vi "Periodic Tasks.vi"(8 "error in":errorcluster) -> ()   [LabVIEW 2015]
doc: "This VI runs in parallel to other tasks. It can contain as many user-defined periodic loops as you need. These can carry out PID or other sorts of timed response."
uses:
  <vilib>/Rock Robotics/WPI/Utilities/WPI_GetSetVariantRefNum.vi
  Robot Global Data.vi
  <vilib>/Rock Robotics/Network Tables/SD Write Boolean.vi
  <vilib>/Rock Robotics/Network Tables/SD Write Number.vi
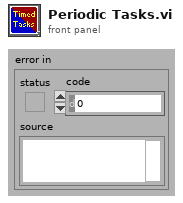
[diagram p1: front panel]
types:
  T1 = typedef "WPI_JoystickDevRef.ctl" = cluster{"Device":T2}
  T2 = typedef "WPI_JoystickDeviceEnum.ctl" = enum16{"USB 0", "USB 1", "USB 2", "USB 3", "USB 4", "USB 5"}
  T3 = cluster{"Axes[0]":dbl, "Axes[1]":dbl, "Axes[2]":dbl, "Axes[3]":dbl, "Axes[4]":dbl, "Axes[5]":dbl, "Axes[6]":dbl, "Axes[7]":dbl, "Axes[8]":dbl}
  T4 = cluster{"Buttons[0]":bool, "Buttons[1]":bool, "Buttons[2]":bool, "Buttons[3]":bool, "Buttons[4]":bool, "Buttons[5]":bool, "Buttons[6]":bool, "Buttons[7]":bool, "Buttons[8]":bool}
  T5 = typedef "WPI_EncoderDevRef.ctl" = cluster{"DevStatus":errorcluster, "EncoderIndex":T6, "CounterIndex":T7, "DistancePerCount":dbl, "Decoding Type":T8}
  T6 = typedef "FPGA_EncoderIdx.ctl" = enum8{"Enc 0", "Enc 1", "Enc 2", "Enc 3", "Enc 4", "Enc 5", "Enc 6", "Enc 7", "Invalid"}
  T7 = typedef "FPGA_CounterCtrSystemIndex.ctl" = enum8{"Ctr 0", "Ctr 1", "Ctr 2", "Ctr 3", "Ctr 4", "Ctr 5", "Ctr 6", "Ctr 7", "Invalid"}
  T8 = typedef "WPI_EncoderType.ctl" = enum16{"1x", "2x", "4x"}
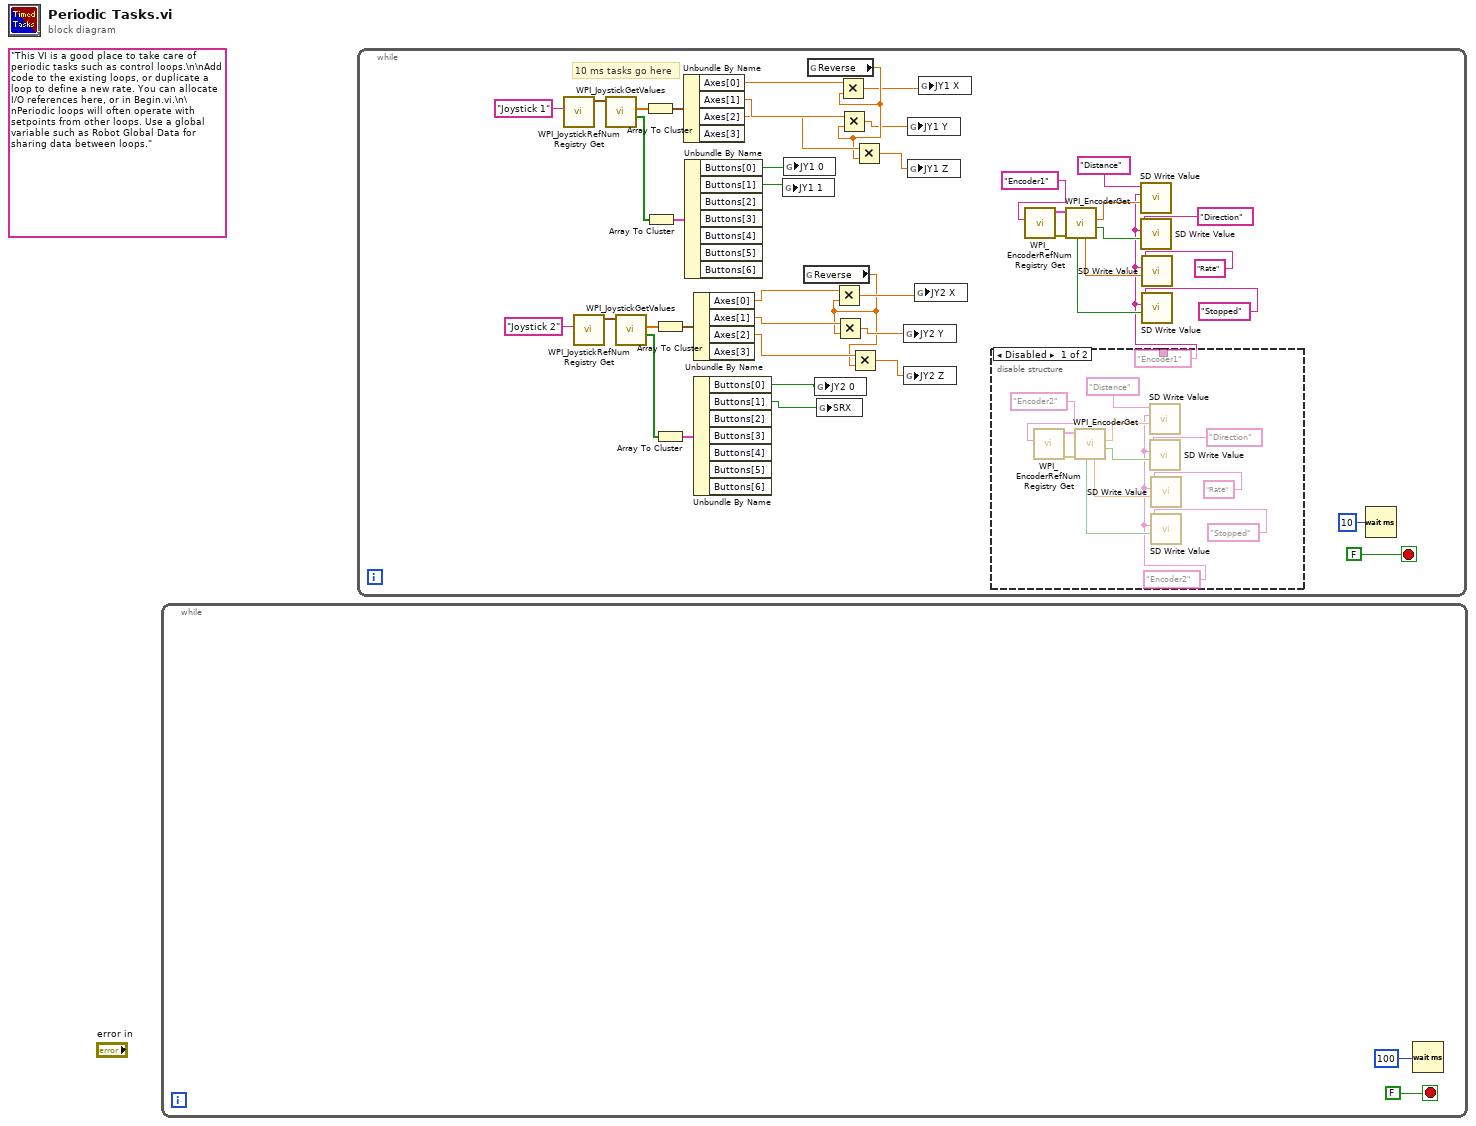
[diagram p0: block diagram]
diagram:
  (unwired) "This VI is a good place to take care of periodic tasks such as control loops.\n\nAdd code to the existing loops, or duplicate a loop to define a new rate. You can allocate I/O references here, or in Begin.vi.\n\nPeriodic loops will often operate with setpoints from other loops. Use a global variable such as Robot Global Data for sharing data between loops."
  n1 = while {
    stop <- FALSE stop-if-true
    n2 = Wait (ms)(milliseconds to wait=u32 100) -> ()  [unwired: 1 out]
  }
  n3 = while {
    stop <- FALSE stop-if-true
    # "10 ms tasks go here"
    n4 = call <vilib>:"WPI_JoystickRefNum Registry Get.vi"("refnum name"="Joystick 1") -> ("JoystickDevRef"=w45:T1)  [unwired: 1 in, 9 out]
    n5 = call <vilib>:"WPI_JoystickRefNum Registry Get.vi"("refnum name"="Joystick 2") -> ("JoystickDevRef"=w39:T1)  [unwired: 1 in, 9 out]
    n6 = call <vilib>:"WPI_JoystickGetValues.vi"("JoystickDevRef"=w45) -> ("Buttons"=w43:bool[], "Axes"=w42:dbl[])  [unwired: 6 in, 3 out]
    n7 = call <vilib>:"WPI_JoystickGetValues.vi"("JoystickDevRef"=w39) -> ("Buttons"=w37:bool[], "Axes"=w36:dbl[])  [unwired: 6 in, 3 out]
    n8 = Array To Cluster(array=w42) -> (cluster=w44:T3)
    n9 = Array To Cluster(array=w43) -> (cluster=w41:T4)
    n10 = Array To Cluster(array=w36) -> (cluster=w38:T3)
    n11 = Array To Cluster(array=w37) -> (cluster=w35:T4)
    n12 = Unbundle By Name(w44) -> ("Axes[0]"=w32:dbl, "Axes[1]"=w31:dbl, "Axes[2]"=w30:dbl)  [unwired: 1 out]
    n13 = Unbundle By Name(w41) -> ("Buttons[0]"=w34:bool, "Buttons[1]"=w33:bool)  [unwired: 5 out]
    n14 = Unbundle By Name(w38) -> ("Axes[0]"=w22:dbl, "Axes[1]"=w21:dbl, "Axes[2]"=w20:dbl)  [unwired: 1 out]
    n15 = Unbundle By Name(w35) -> ("Buttons[0]"=w18:bool, "Buttons[1]"=w3:bool)  [unwired: 5 out]
    n16 = global write "Robot Global Data.vi" "JY1 1"(w33) -> ()
    n17 = global write "Robot Global Data.vi" "JY1 0"(w34) -> ()
    n18 = global read "Robot Global Data.vi" "Reverse"() -> (w19:dbl)
    n19 = global read "Robot Global Data.vi" "Reverse"() -> (w29:dbl)
    n20 = global write "Robot Global Data.vi" "JY2 0"(w18) -> ()
    n21 = global write "Robot Global Data.vi" "SRX"(w3) -> ()
    n22 = Multiply(x=w22, y=w19) -> (x*y=w25:dbl)
    n23 = Multiply(x=w21, y=w19) -> (x*y=w24:dbl)
    n24 = Multiply(x=w32, y=w29) -> (x*y=w28:dbl)
    n25 = Multiply(x=w31, y=w29) -> (x*y=w27:dbl)
    n26 = Multiply(x=w20, y=w19) -> (x*y=w23:dbl)
    n27 = Multiply(x=w30, y=w29) -> (x*y=w26:dbl)
    n28 = global write "Robot Global Data.vi" "JY2 Y"(w24) -> ()
    n29 = global write "Robot Global Data.vi" "JY2 Z"(w23) -> ()
    n30 = global write "Robot Global Data.vi" "JY1 Y"(w27) -> ()
    n31 = global write "Robot Global Data.vi" "JY1 Z"(w26) -> ()
    n32 = global write "Robot Global Data.vi" "JY2 X"(w25) -> ()
    n33 = global write "Robot Global Data.vi" "JY1 X"(w28) -> ()
    n34 = disable-structure shown="Disabled" {
      disable-tunnel: ["Encoder1" _] -> w6
      frame Disabled {
        w47 = "Encoder2"
        n35 = call <vilib>:"WPI_EncoderRefNum Registry Get.vi"("refnum name"="Encoder2") -> ("error out"=w58:errorcluster, "EncoderDevRef"=w57:T5)  [unwired: 9 in]
        n36 = call <vilib>:"WPI_EncoderGet.vi"("error in (no error)"=w58, "EncoderDevRef"=w57) -> ("Direction"=w54:bool, "Distance"=w55:dbl, "Rate"=w53:dbl, "Stopped"=w52:bool)  [unwired: 4 in, 2 out]
        n37 = call-poly <vilib>:"SD Write Value.vi"("Numeric"=w55, "Table Prefix"=w47, "Name"="Distance") -> ()  [unwired: 7 in, 2 out]
        n38 = call-poly <vilib>:"SD Write Value.vi"("Boolean"=w54, "Table Prefix"=w47, "Name"="Direction") -> ()  [unwired: 7 in, 2 out]
        n39 = call-poly <vilib>:"SD Write Value.vi"("Numeric"=w53, "Table Prefix"=w47, "Name"="Rate") -> ()  [unwired: 7 in, 2 out]
        n40 = call-poly <vilib>:"SD Write Value.vi"("Boolean"=w52, "Table Prefix"=w47, "Name"="Stopped") -> ()  [unwired: 7 in, 2 out]
      }
      frame Enabled {
      }
    }
    n41 = call <vilib>:"WPI_EncoderRefNum Registry Get.vi"("refnum name"="Encoder1") -> ("error out"=w17:errorcluster, "EncoderDevRef"=w16:T5)  [unwired: 9 in]
    n42 = call <vilib>:"WPI_EncoderGet.vi"("error in (no error)"=w17, "EncoderDevRef"=w16) -> ("Direction"=w13:bool, "Distance"=w14:dbl, "Rate"=w12:dbl, "Stopped"=w11:bool)  [unwired: 4 in, 2 out]
    n43 = call-poly <vilib>:"SD Write Value.vi"("Numeric"=w14, "Table Prefix"=w6, "Name"="Distance") -> ()  [unwired: 7 in, 2 out]
    n44 = call-poly <vilib>:"SD Write Value.vi"("Boolean"=w13, "Table Prefix"=w6, "Name"="Direction") -> ()  [unwired: 7 in, 2 out]
    n45 = call-poly <vilib>:"SD Write Value.vi"("Numeric"=w12, "Table Prefix"=w6, "Name"="Rate") -> ()  [unwired: 7 in, 2 out]
    n46 = call-poly <vilib>:"SD Write Value.vi"("Boolean"=w11, "Table Prefix"=w6, "Name"="Stopped") -> ()  [unwired: 7 in, 2 out]
    n47 = Wait (ms)(milliseconds to wait=u32 10) -> ()  [unwired: 1 out]
  }
